vi "Meas - Send Meas VI Names.vi"(8 "Error In":errorcluster) -> (0 "Error Out":errorcluster)   [LabVIEW 2011]
doc: "This VI will send the Meas VI name to the MEAS_LIST queue."
uses:
  Controls/INIT- READ - WRITE.ctl
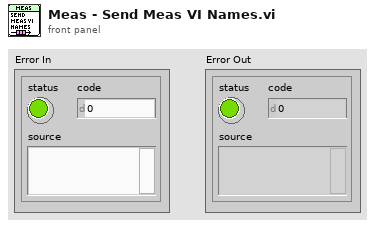
[diagram p1: front panel]
types:
  T1 = typedef "INIT- READ - WRITE.ctl" = enum16{"INIT", "READ", "WRITE"}
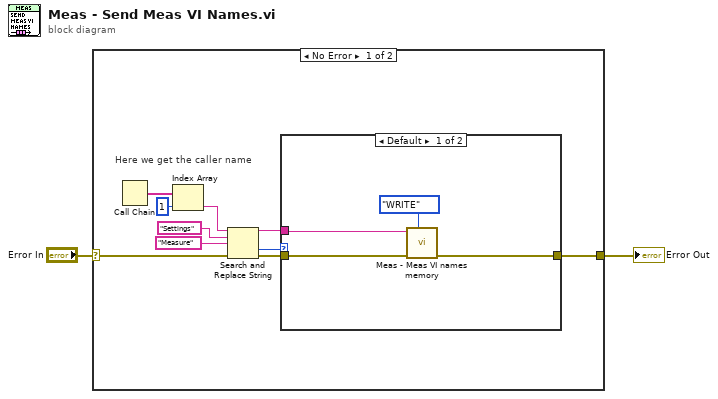
[diagram p0: block diagram]
diagram:
  n1 = case shown="No Error" "Error In" {
    selector: "Error In" -> [w3 w18]
    tunnel: [w4 w18] -> w2
    frame No Error {
      # "Here we get the caller name"
      n2 = Call Chain() -> (call chain=w12:string[])
      n3 = Index Array(array=w12, index=1) -> (element=w10:string)
      n4 = Search and Replace String(input string=w10, search string="Settings", replace string="Measure" ("search string"), error in=w3) -> (result string=w6:string, offset past replacement=w7:i32, error out=w5:errorcluster)  [unwired: 4 in, 1 out]
      n5 = case shown="Default" w7 {
        tunnel: w6 -> [w14 _]
        tunnel: w5 -> [w16 w17]
        tunnel: [w15 w17] -> w4
        frame Default {
          n6 = call "Meas - Meas VI names memory.vi"("Operation"=INIT-_READ_-_WRITE."WRITE", "Error In"=w16, "Name In"=w14) -> ("Error Out"=w15:errorcluster)  [unwired: 7 in, 1 out]
        }
        frame -1 {
        }
      }
    }
    frame Error {
    }
  }
  "Error Out" <- w2
